vi "myRIO_BRig_RT__Case_Exp_subState_LC__initTrial.vi"(6 "input_dataTrial":u16[][](array[numeric]), 7 "input_spout":enum16{"Left", "Right"}(ring), 8 "input_dataCurrent":u16[](array[numeric]), 10 "input_dataLC":u16[](array[numeric])) -> (0 "output_LC_Wrong":bool, 1 "output_LC_led_Wrong":bool, 2 "output_LC_Reward":bool, 3 "output_LC_led_Reward":bool, 4 "output_dataTrial":u16[][](array[numeric]))   [LabVIEW 2014]
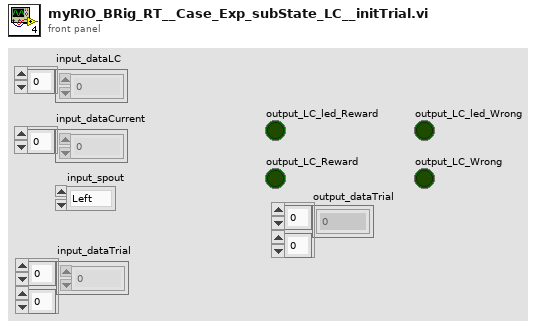
[diagram p1: front panel]
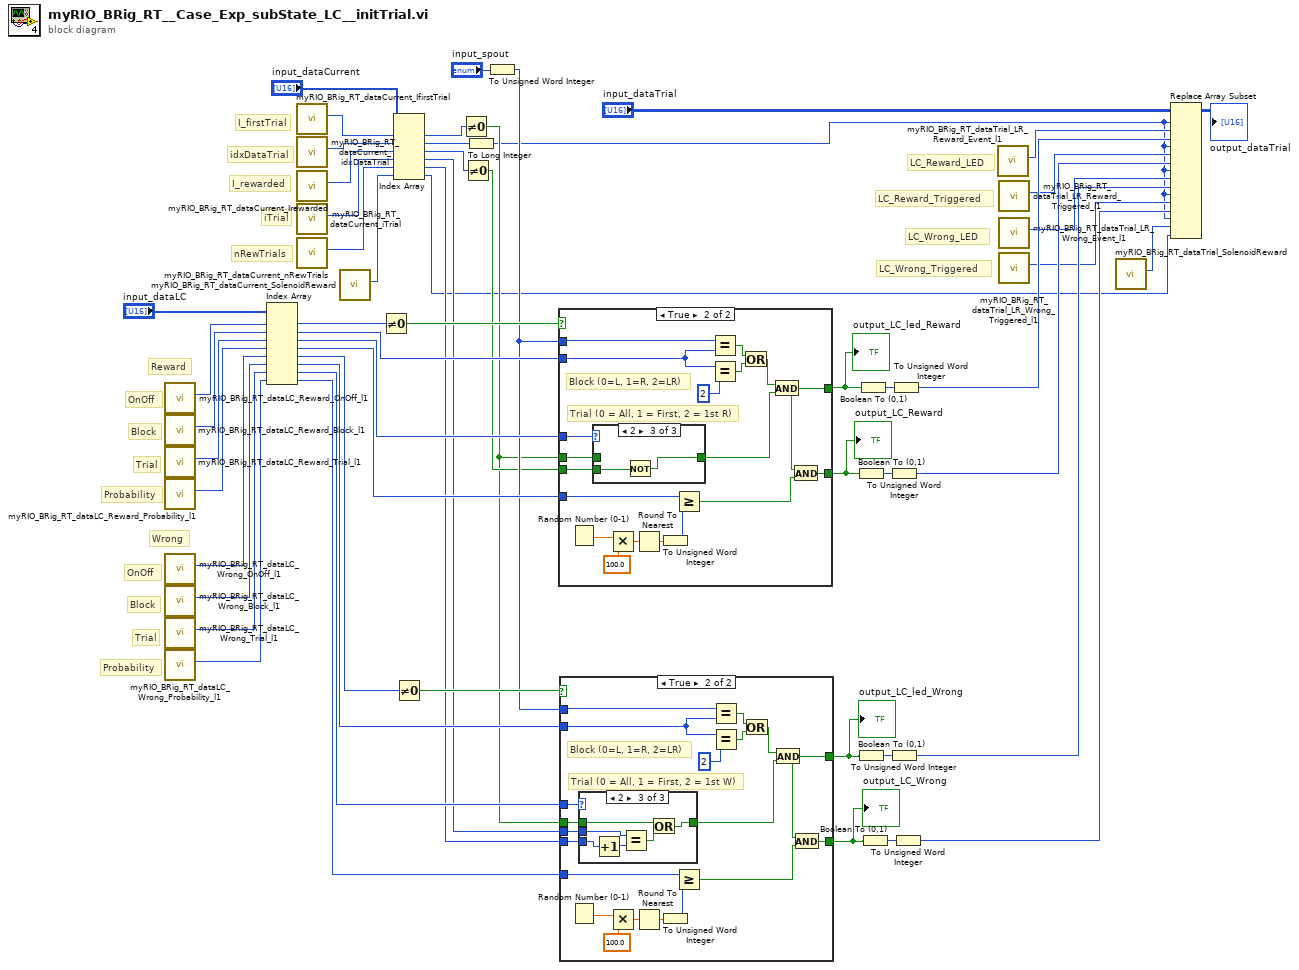
[diagram p0: block diagram]
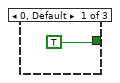
[diagram p3: hidden frame]
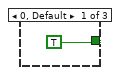
[diagram p6: hidden frame]
diagram:
  # "nRewTrials"
  # "iTrial"
  # "I_rewarded"
  # "LC_Wrong_Triggered"
  # "LC_Wrong_LED"
  # "LC_Reward_Triggered"
  # "LC_Reward_LED"
  # "idxDataTrial"
  # "Probability"
  # "Trial"
  # "Block"
  # "OnOff"
  # "Wrong"
  # "I_firstTrial"
  # "Reward"
  # "Probability"
  # "Trial"
  # "Block"
  # "OnOff"
  n1 = call "myRIO_BRig_RT_dataLC_Reward_OnOff_l1.vi"() -> ("output_Reward_OnOff_l1"=w55:i32)  [unwired: 11 in]
  n2 = call "myRIO_BRig_RT_dataLC_Reward_Block_l1.vi"() -> ("output_Reward_Block_l1"=w54:i32)  [unwired: 11 in]
  n3 = call "myRIO_BRig_RT_dataLC_Reward_Trial_l1.vi"() -> ("output_Reward_Trial_l1"=w53:i32)  [unwired: 11 in]
  n4 = call "myRIO_BRig_RT_dataLC_Reward_Probability_l1.vi"() -> ("output_Reward_Probability_l1"=w52:i32)  [unwired: 11 in]
  n5 = call "myRIO_BRig_RT_dataLC_Wrong_OnOff_l1.vi"() -> ("output_Wrong_OnOff_l1"=w40:i32)  [unwired: 11 in]
  n6 = call "myRIO_BRig_RT_dataLC_Wrong_Block_l1.vi"() -> ("output_Wrong_Block_l1"=w41:i32)  [unwired: 11 in]
  n7 = call "myRIO_BRig_RT_dataLC_Wrong_Trial_l1.vi"() -> ("output_Wrong_Trial_l1"=w42:i32)  [unwired: 11 in]
  n8 = call "myRIO_BRig_RT_dataLC_Wrong_Probability_l1.vi"() -> ("output_Wrong_Probability_l1"=w43:i32)  [unwired: 11 in]
  n9 = Index Array(array="input_dataLC", index #1=w55, index #2=w54, index #3=w53, index #4=w52, index #5=w40, index #6=w41, index #7=w42, index #8=w43) -> (element #1=w51:u16, element #2=w49:u16, element #3=w48:u16, element #4=w47:u16, element #5=w37:u16, element #6=w35:u16, element #7=w34:u16, element #8=w33:u16)
  n10 = call "myRIO_BRig_RT_dataCurrent_IfirstTrial.vi"() -> ("output_I_firstTrial"=w45:i32)  [unwired: 11 in]
  n11 = call "myRIO_BRig_RT_dataCurrent_idxDataTrial.vi"() -> ("output_idxDataTrial"=w32:i32)  [unwired: 11 in]
  n12 = call "myRIO_BRig_RT_dataCurrent_Irewarded.vi"() -> ("output_I_rewarded"=w12:i32)  [unwired: 11 in]
  n13 = call "myRIO_BRig_RT_dataCurrent_iTrial.vi"() -> ("output_iTrial"=w10:i32)  [unwired: 11 in]
  n14 = call "myRIO_BRig_RT_dataCurrent_nRewTrials.vi"() -> ("output_nRewTrials"=w7:i32)  [unwired: 11 in]
  n15 = call "myRIO_BRig_RT_dataCurrent_SolenoidReward.vi"() -> ("output_SolenoidReward"=w4:i32)  [unwired: 11 in]
  n16 = Not Equal To 0?(x=w51) -> (x != 0?=w50:bool)
  n17 = Index Array(array="input_dataCurrent", index #1=w45, index #2=w32, index #3=w12, index #4=w10, index #5=w7, index #6=w4) -> (element #1=w44:u16, element #2=w31:u16, element #3=w11:u16, element #4=w9:u16, element #5=w6:u16, element #6=w1:u16)
  n18 = Not Equal To 0?(x=w37) -> (x != 0?=w38:bool)
  n19 = Not Equal To 0?(x=w44) -> (x != 0?=w5:bool)
  n20 = Not Equal To 0?(x=w11) -> (x != 0?=w8:bool)
  n21 = To Long Integer(number=w31) -> (32bit integer=w3:i32)
  n22 = To Unsigned Word Integer(number="input_spout") -> (unsigned 16bit integer=w36:u16)
  n23 = case shown="True" w50 {
    tunnel: w49 -> [_ w66]
    tunnel: w48 -> [_ w60]
    tunnel: w47 -> [_ w67]
    tunnel: [_ w63] -> w23
    tunnel: [_ w62] -> w27
    tunnel: w36 -> [_ w61]
    tunnel: w8 -> [_ w57]
    tunnel: w5 -> [_ w59]
    frame False {
    }
    frame True {
      # "Block (0=L, 1=R, 2=LR)"
      # "Trial (0 = All, 1 = First, 2 = 1st R)"
      n24 = Random Number (0-1)() -> (number: 0 to 1=w72:dbl)
      n25 = case shown="2" w60 {
        tunnel: w59 -> [_ w77 _]
        tunnel: [TRUE w77 w78] -> w58
        tunnel: w57 -> [_ _ w79]
        frame 0, Default {
        }
        frame 1 {
        }
        frame 2 {
          n26 = Not(x=w79) -> (.not. x?=w78:bool)
        }
      }
      n27 = Multiply(x=w72, y=100.0) -> (x*y=w71:dbl)
      n28 = Round To Nearest(number=w71) -> (nearest integer value=w70:dbl)
      n29 = To Unsigned Word Integer(number=w70) -> (unsigned 16bit integer=w69:u16)
      n30 = Greater Or Equal?(x=w67, y=w69) -> (x >= y?=w65:bool)
      n31 = Equal?(x=w61, y=w66) -> (x = y?=w74:bool)
      n32 = Equal?(x=w66, y=u16 2) -> (x = y?=w73:bool)
      n33 = Or(x=w74, y=w73) -> (x .or. y?=w64:bool)
      n34 = And(x=w64, y=w58) -> (x .and. y?=w62:bool)
      n35 = And(x=w62, y=w65) -> (x .and. y?=w63:bool)
    }
  }
  "output_LC_Reward" <- w23
  "output_LC_led_Reward" <- w27
  n36 = case shown="True" w38 {
    tunnel: w35 -> [_ w90]
    tunnel: w34 -> [_ w84]
    tunnel: w33 -> [_ w91]
    tunnel: [_ w87] -> w14
    tunnel: [_ w86] -> w18
    tunnel: w36 -> [_ w85]
    tunnel: w5 -> [_ w82]
    tunnel: w9 -> [_ w81]
    tunnel: w6 -> [_ w80]
    frame False {
    }
    frame True {
      # "Block (0=L, 1=R, 2=LR)"
      # "Trial (0 = All, 1 = First, 2 = 1st W)"
      n37 = Random Number (0-1)() -> (number: 0 to 1=w96:dbl)
      n38 = case shown="2" w84 {
        tunnel: [TRUE w101 w106] -> w83
        tunnel: w82 -> [_ w101 w107]
        tunnel: w81 -> [_ _ w103]
        tunnel: w80 -> [_ _ w105]
        frame 0, Default {
        }
        frame 1 {
        }
        frame 2 {
          n39 = Increment(x=w105) -> (x+1=w104:u16)
          n40 = Equal?(x=w103, y=w104) -> (x = y?=w102:bool)
          n41 = Or(x=w107, y=w102) -> (x .or. y?=w106:bool)
        }
      }
      n42 = Multiply(x=w96, y=100.0) -> (x*y=w95:dbl)
      n43 = Round To Nearest(number=w95) -> (nearest integer value=w94:dbl)
      n44 = To Unsigned Word Integer(number=w94) -> (unsigned 16bit integer=w93:u16)
      n45 = Greater Or Equal?(x=w91, y=w93) -> (x >= y?=w89:bool)
      n46 = Equal?(x=w85, y=w90) -> (x = y?=w98:bool)
      n47 = Equal?(x=w90, y=u16 2) -> (x = y?=w97:bool)
      n48 = Or(x=w98, y=w97) -> (x .or. y?=w88:bool)
      n49 = And(x=w88, y=w83) -> (x .and. y?=w86:bool)
      n50 = And(x=w86, y=w89) -> (x .and. y?=w87:bool)
    }
  }
  "output_LC_Wrong" <- w14
  "output_LC_led_Wrong" <- w18
  n51 = Boolean To (0,1)(Boolean=w23) -> (0, 1=w24:i16)
  n52 = Boolean To (0,1)(Boolean=w18) -> (0, 1=w19:i16)
  n53 = Boolean To (0,1)(Boolean=w27) -> (0, 1=w26:i16)
  n54 = Boolean To (0,1)(Boolean=w14) -> (0, 1=w15:i16)
  n55 = To Unsigned Word Integer(number=w24) -> (unsigned 16bit integer=w21:u16)
  n56 = To Unsigned Word Integer(number=w19) -> (unsigned 16bit integer=w17:u16)
  n57 = To Unsigned Word Integer(number=w26) -> (unsigned 16bit integer=w25:u16)
  n58 = To Unsigned Word Integer(number=w15) -> (unsigned 16bit integer=w13:u16)
  n59 = call "myRIO_BRig_RT_dataTrial_LR_Reward_Event_l1.vi"() -> ("output_LR_Reward_Event_l1"=w28:i32)  [unwired: 11 in]
  n60 = call "myRIO_BRig_RT_dataTrial_LR_Reward_Triggered_l1.vi"() -> ("output_LR_Reward_Triggered_l1"=w22:i32)  [unwired: 11 in]
  n61 = call "myRIO_BRig_RT_dataTrial_LR_Wrong_Event_l1.vi"() -> ("output_LR_Wrong_Event_l1"=w20:i32)  [unwired: 11 in]
  n62 = call "myRIO_BRig_RT_dataTrial_LR_Wrong_Triggered_l1.vi"() -> ("output_LR_Wrong_Triggered_l1"=w16:i32)  [unwired: 11 in]
  n63 = call "myRIO_BRig_RT_dataTrial_SolenoidReward.vi"() -> ("output_SolenoidReward"=w2:i32)  [unwired: 11 in]
  n64 = Replace Array Subset(array="input_dataTrial", new element #1=w25, index (row) #1=w3, index (col) #1=w28, new element #2=w21, index (row) #2=w3, index (col) #2=w22, new element #3=w17, index (row) #3=w3, index (col) #3=w20, new element #4=w13, index (row) #4=w3, index (col) #4=w16, new element #5=w1, index (row) #5=w3, index (col) #5=w2) -> (→"output_dataTrial":u16[][])
